vi "Get Yaw.vi"() -> (0 "Angle":dbl)   [LabVIEW 2017]
uses:
  Robot Global Data.vi
  <vilib>/Rock Robotics/WPI/ThirdParty/Phoenix-LabVIEW/Pigeon IMU/CTRE_PigeonIMU_GetYPR.vi
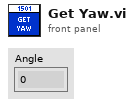
[diagram p1: front panel]
types:
  T1 = typedef "CTRE_PigeonIMU_DeviceRef.ctl" = cluster{"DeviceStatus":errorcluster, "Device Number":u8, "Type":T2, "Device ID":u32, "Handle":u64, "UsageFrame":u32, "Library Path":path}
  T2 = typedef "CTRE_PigeonIMU_ConnectionType.ctl" = u32
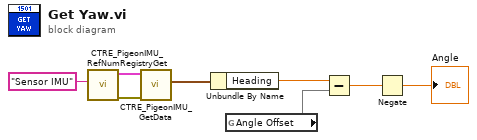
[diagram p0: block diagram]
diagram:
  n1 = call <vilib>:"CTRE_PigeonIMU_RefNumRegistryGet.vi"("refnum name"="Sensor IMU") -> ("error out"=w6:errorcluster, "PigeonIMUDevRef"=w7:T1)  [unwired: 9 in]
  n2 = call-poly <vilib>:"CTRE_PigeonIMU_GetData.vi"("error in (no error)"=w6, "PigeonIMUDevRef"=w7) -> ("Yaw Pitch Roll"=w3:cluster{"Yaw":dbl, "Pitch":dbl, "Roll":dbl})  [unwired: 7 in, 2 out]
  n3 = Unbundle By Name(w3) -> ("Heading"=w2:dbl)
  n4 = global read "Robot Global Data.vi" "Angle Offset"() -> (w4)
  n5 = Subtract(x=w2, y=w4) -> (x-y=w5:dbl)
  n6 = Negate(x=w5) -> (-x=→"Angle":dbl)
